vi "Subscribe.vi"(8 "error in (no error)":errorcluster, 9 "Name":string, 10 "Receivers Enqueuer":refnum<class "Message Enqueuer.lvclass">, 11 "Pub Sub Retaining Message Channel in":refnum<class "Pub Sub Retaining Message Channel.lvclass">) -> (0 "error out":errorcluster, 2 "New Subscription":bool, 3 "Pub Sub Retaining Message Channel out":refnum<class "Pub Sub Retaining Message Channel.lvclass">)   [LabVIEW 2020, in "Actor Pub Sub Channels.lvlib" / "Pub Sub Retaining Message Channel.lvclass"]
uses:
  Pub Sub Retaining Message Channel.lvclass
  <vilib>/ActorFramework/Message Enqueuer/Message Enqueuer.lvclass
  <vilib>/ActorFramework/Message/Message.lvclass
  Pub Sub Retaining Message Channel.lvclass/Pub Sub Retaining Message Channel.ctl
  <vilib>/ActorFramework/Self-Addressed Msg/Self-Addressed Msg.lvclass
  Pub Sub Message Channel/Pub Sub Message Channel.lvclass
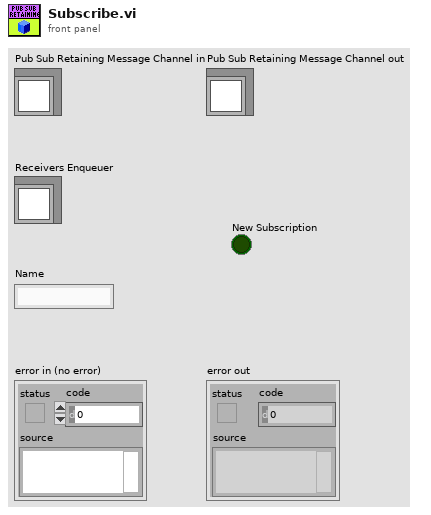
[diagram p1: front panel]
types:
  T1 = cluster{"Actor Framework:Message":refnum<class "Message.lvclass">}
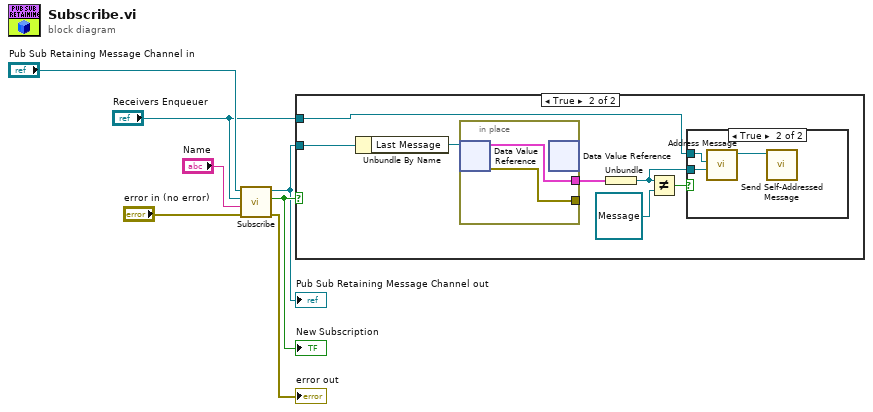
[diagram p0: block diagram]
diagram:
  n1 = call-parent "Subscribe.vi"("error in (no error)"="error in (no error)", "Name"="Name", "Receivers Enqueuer"="Receivers Enqueuer", "Pub Sub Message Channel in"="Pub Sub Retaining Message Channel in") -> ("error out"=→"error out":errorcluster, "New Subscription"=w3:bool, "Pub Sub Message Channel out"=w2:refnum<class "Pub Sub Retaining Message Channel.lvclass">)  [unwired: 5 in]
  "Pub Sub Retaining Message Channel out" <- w2
  "New Subscription" <- w3
  n2 = case shown="True" w3 {
    tunnel: w2 -> [_ w14]
    tunnel: "Receivers Enqueuer" -> [_ w10]
    frame False {
    }
    frame True {
      n3 = Unbundle By Name(w14) -> ("Last Message"=w13:refnum<data-value>)
      n4 = in-place {
        in-place-border: [w19] -> w12
        in-place-border: [w18] -> _
        n5 = in-place-dvr #1(w13) -> (w19:T1, w18:errorcluster)
        n6 = in-place-dvr #1() -> ()  [unwired: 1 in, 2 out]
      }
      n7 = Unbundle(w12) -> ("Actor Framework:Message"=w8:refnum<class "Message.lvclass">)
      n8 = Not Equal?(x=w8, y=refnum<class "Message.lvclass"> refnum) -> (x != y?=w9:bool)
      n9 = case shown="True" w9 {
        tunnel: w10 -> [_ w17]
        tunnel: w8 -> [_ w16]
        frame False {
        }
        frame True {
          n10 = call <vilib>:"Address Message.vi"("Message"=w16, "Destination"=w17) -> ("Self-Addressed Message"=w15:refnum<class "Self-Addressed Msg.lvclass">)  [unwired: 9 in]
          n11 = call-dynamic "Send Self-Addressed Message.vi"("Self-Addressed Message in"=w15) -> ()  [unwired: 9 in, 2 out]
        }
      }
    }
  }
